vi "Offset Widget Offset Values.vi"(7 "Force Offset Tag":string, 8 "Coordinate Space":bool caption="Coord", 9 "Rigid Connection In":bool, 10 "Number of\nLBCBs":T1, 11 "Offset Type":T2) -> (3 "Offsets":dbl[][](array[numeric]))   [LabVIEW 2009]
uses:
  Offset Types.ctl
  Data Access Objects/Application/Number Of LBCBs.ctl
  Global Data/Dataset Transaction Id.ctl
  Global Data/Dataset Source.ctl
  Global Data/Dataset Type.ctl
  Apps/Yes No Button.ctl
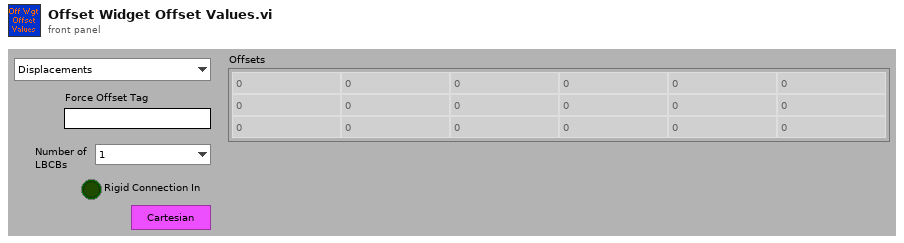
[diagram p1: front panel]
types:
  T1 = typedef "Number Of LBCBs.ctl" = enum16{"1", "2"}
  T2 = typedef "Offset Types.ctl" = enum16{"Displacements", "Forces", "External Sensors"}
  T3 = typedef "Dataset Transaction Id.ctl" = cluster{"Dataset Source":T4, "Dataset Type":T5, "Hold":T6, "Volts":T6, "Tag":string}
  T4 = typedef "Dataset Source.ctl" = enum16{"LBCB 1", "LBCB 2", "Combined", "External Sensors"}
  T5 = typedef "Dataset Type.ctl" = enum16{"LVDT", "Load Cell", "Actuator Command", "Servo Error", "Displacement Command", "Displacement", "Force"}
  T6 = typedef "Yes No Button.ctl" = bool
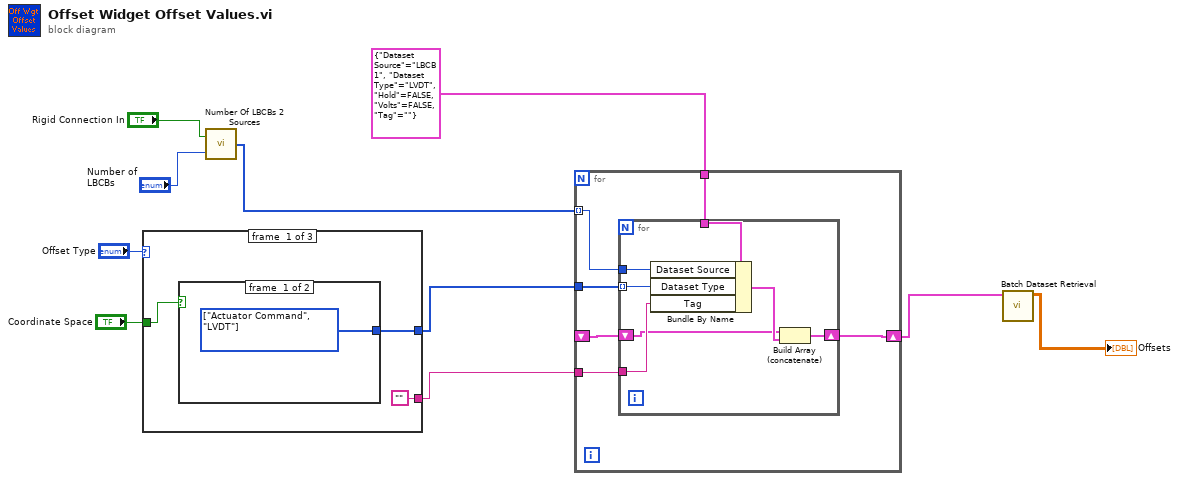
[diagram p0: block diagram]
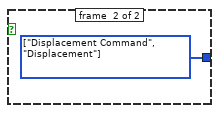
[diagram p2: hidden frame]
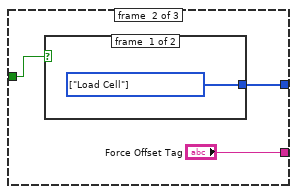
[diagram p3: hidden frame]
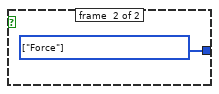
[diagram p4: hidden frame]
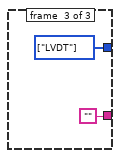
[diagram p5: hidden frame]
diagram:
  n1 = case shown="\"Displacements\"" "Offset Type" {
    tunnel: "Coordinate Space" -> [w13 w18 _]
    tunnel: [w12 w17 w22] -> w4
    tunnel: ["" "Force Offset Tag" ""] -> w1
    frame #0 {
      n2 = case shown="False" w13 {
        tunnel: [w14 w15] -> w12
        frame #0 {
          w14 = T5[] [enum."Actuator Command", enum."LVDT"] items=["LVDT", "Load Cell", "Actuator Command", "Servo Error", "Displacement Command", "Displacement", "Force"]
        }
        frame #1 {
          w15 = T5[] [enum."Displacement Command", enum."Displacement"] items=["LVDT", "Load Cell", "Actuator Command", "Servo Error", "Displacement Command", "Displacement", "Force"]
        }
      }
    }
    frame #1 {
      n3 = case shown="True" w18 {
        tunnel: [w19 w20] -> w17
        frame #0 {
          w19 = T5[] [enum."Load Cell"] items=["LVDT", "Load Cell", "Actuator Command", "Servo Error", "Displacement Command", "Displacement", "Force"]
        }
        frame #1 {
          w20 = T5[] [enum."Force"] items=["LVDT", "Load Cell", "Actuator Command", "Servo Error", "Displacement Command", "Displacement", "Force"]
        }
      }
    }
    frame #2 {
      w22 = T5[] [enum."LVDT"] items=["LVDT", "Load Cell", "Actuator Command", "Servo Error", "Displacement Command", "Displacement", "Force"]
    }
  }
  n4 = call "Number Of LBCBs 2 Sources.vi"("Number of LBCBs"="Number of\nLBCBs", "Combined LBCBs"="Rigid Connection In") -> ("Sources"=w8:T4[])
  n5 = for {
    tunnel: w8 -> [w26] mode=indexing
    tunnel: T3 {"Dataset Source"=enum."LBCB 1", "Dataset Type"=enum."LVDT", "Hold"=FALSE, "Volts"=FALSE, "Tag"=""} ("Dataset Trans Id") -> [w28]
    tunnel: w1 -> [w27]
    tunnel: w4 -> [w25]
    shift-right: [w24] -> w3
    shift-left: _ -> [w23]
    n6 = for {
      tunnel: w28 -> [w35]
      tunnel: w27 -> [w34]
      tunnel: w26 -> [w33]
      tunnel: w25 -> [w32] mode=indexing
      shift-right: [w30] -> w24
      shift-left: w23 -> [w29]
      n7 = Bundle By Name(cluster=w35, "Dataset Source"=w33, "Dataset Type"=w32, "Tag"=w34) -> (w31:T3)
      n8 = Build Array (concatenate)(w29, w31) -> (w30:T3[])
    }
  }
  n9 = call "Batch Dataset Retrieval.vi"("Transactions"=w3) -> ("Data"=→"Offsets":dbl[][])  [unwired: 9 in, 1 out]
